vi "5.6.vi"() -> ()   [LabVIEW 2016]
uses:
  <vilib>/sound2/lvsound2.llb/Sound Data Format.ctl
  <vilib>/Analysis/4window.llb/Hamming Window (DBL).vi
  <vilib>/Analysis/2dsp.llb/Real FFT.vi
  <vilib>/Analysis/4window.llb/AllCosWindow (DBL).vi
  <vilib>/sound2/lvsound2.llb/Sound File Info (path).vi
  <vilib>/Analysis/3filter.llb/Butterworth Filter (DBL).vi
  <vilib>/Analysis/NI_AALPro.lvlib
  <vilib>/Analysis/NI_AALBase.lvlib
panel:
  out "count":i32
  out "differentiator output":dbl[](graph)
  out "comparator output":dbl[](graph)
  in  "threshold2":dbl
  out "envelope detector output":dbl[](graph)
  out "All":waveform(dbl)(graph)
  in  "Length":dbl(slide) scale=0.0..1024.0
  out "D":bool
  out "#":bool
  out "0":bool
  out "*":bool
  out "C":bool
  out "9":bool
  out "8":bool
  out "7":bool
  out "B":bool
  out "6":bool
  out "5":bool
  out "4":bool
  out "A":bool
  out "3":bool
  out "2":bool
  out "1":bool
  in  "Threshold":dbl
  out "Sub":waveform(dbl)(graph)
  out "FFT":dbl[](graph)
  out "sampling reate":dbl
  out "sound format":T1={"sample rate (S/s)"=22050.0, "number of channels"=2, "bits per sample"=16}
  in  "Path":path
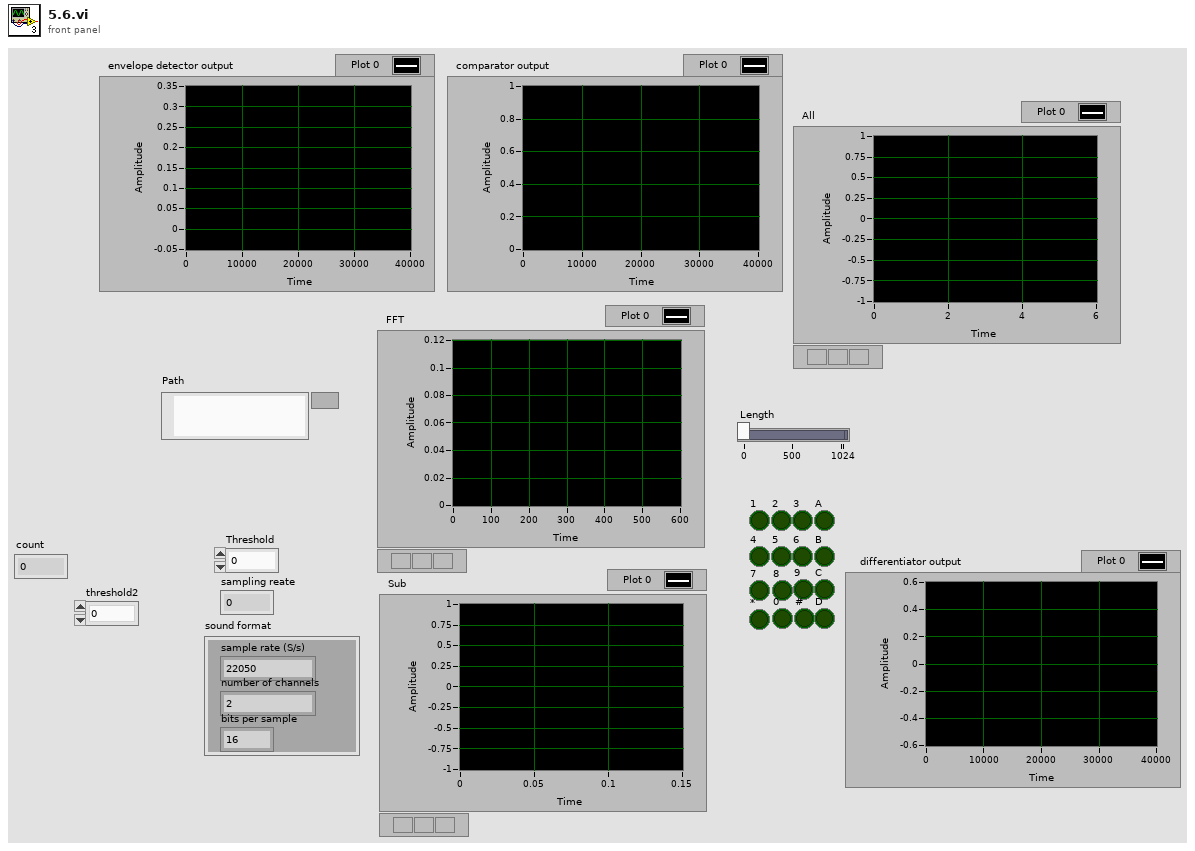
[diagram p1: front panel]
types:
  T1 = typedef "Sound Data Format.ctl" = cluster{"sample rate (S/s)":dbl, "number of channels":i32, "bits per sample":i32}
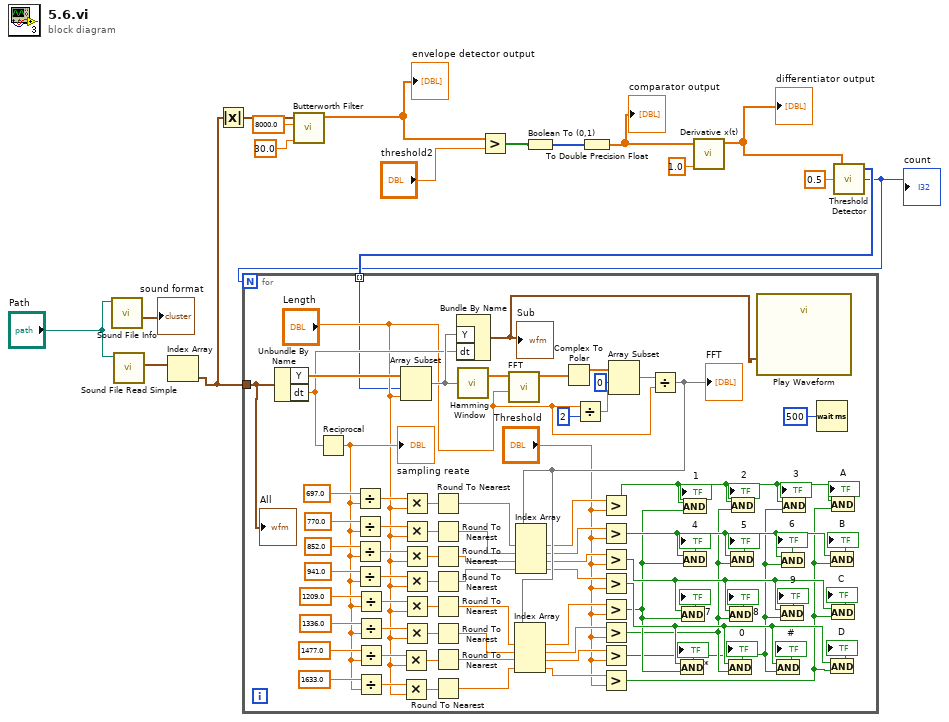
[diagram p0: block diagram]
diagram:
  n1 = call-poly <vilib>:"Sound File Info.vi"("path"="Path") -> ("sound format"=→"sound format":T1)  [unwired: 7 in, 3 out]
  n2 = call <vilib>:"Sound File Read Simple.vi"("path"="Path") -> ("data"=w17:waveform(dbl)[])  [unwired: 7 in, 3 out]
  n3 = Index Array(array=w17) -> (element=w3:waveform(dbl))  [unwired: 1 in]
  n4 = Absolute Value(x=w3) -> (abs(x)=w5:waveform(dbl))
  n5 = call-poly <vilib>:"Butterworth Filter.vi"("low cutoff freq: fl"=30.0, "sampling freq: fs"=8000.0, "X"=w5) -> ("Filtered X"=w13:dbl[])  [unwired: 5 in, 1 out]
  "envelope detector output" <- w13
  n6 = Greater?(x=w13, y="threshold2") -> (0:w11:bool[])
  n7 = Boolean To (0,1)(Boolean=w11) -> (0, 1=w10:i16[])
  n8 = To Double Precision Float(number=w10) -> (double precision float=w9:dbl[])
  "comparator output" <- w9
  n9 = call <vilib>:"Derivative x(t).vi"("dt"=1.0, "X"=w9) -> ("dX/dt"=w7:dbl[])  [unwired: 8 in, 1 out]
  "differentiator output" <- w7
  n10 = call <vilib>:"Threshold Detector.vi"("threshold"=0.5, "X"=w7) -> ("count"=w1:i32, "Indices"=w2:i32[])  [unwired: 1 in, 1 out]
  "count" <- w1
  n11 = for {
    N: w1 -> [_]
    tunnel: w3 -> [w22]
    tunnel: w2 -> [w19] mode=indexing
    n12 = Unbundle By Name(w22) -> ("Y"=w99:dbl[], "dt"=w74:dbl)
    n13 = Reciprocal(x=w74) -> (1/x=w82:dbl)
    "sampling reate" <- w82
    n14 = Divide(x=697.0, y=w82) -> (x/y=w83:dbl)
    n15 = Divide(x=770.0, y=w82) -> (x/y=w84:dbl)
    n16 = Divide(x=852.0, y=w82) -> (x/y=w85:dbl)
    n17 = Divide(x=941.0, y=w82) -> (x/y=w86:dbl)
    n18 = Divide(x=1209.0, y=w82) -> (x/y=w87:dbl)
    n19 = Divide(x=1336.0, y=w82) -> (x/y=w88:dbl)
    n20 = Divide(x=1477.0, y=w82) -> (x/y=w89:dbl)
    n21 = Divide(x=1633.0, y=w82) -> (x/y=w90:dbl)
    n22 = Array Subset(array=w99, index=w19, length="Length") -> (w75:dbl[])
    n23 = Multiply(x=w89, y="Length") -> (x*y=w67:dbl)
    n24 = Multiply(x=w90, y="Length") -> (x*y=w66:dbl)
    n25 = Multiply(x=w83, y="Length") -> (x*y=w73:dbl)
    n26 = Multiply(x=w84, y="Length") -> (x*y=w72:dbl)
    n27 = Multiply(x=w85, y="Length") -> (x*y=w71:dbl)
    n28 = Multiply(x=w86, y="Length") -> (x*y=w70:dbl)
    n29 = Multiply(x=w87, y="Length") -> (x*y=w69:dbl)
    n30 = Multiply(x=w88, y="Length") -> (x*y=w68:dbl)
    n31 = Round To Nearest(number=w73) -> (nearest integer value=w65:dbl)
    n32 = Round To Nearest(number=w72) -> (nearest integer value=w64:dbl)
    n33 = Round To Nearest(number=w71) -> (nearest integer value=w63:dbl)
    n34 = Round To Nearest(number=w70) -> (nearest integer value=w62:dbl)
    n35 = Round To Nearest(number=w69) -> (nearest integer value=w61:dbl)
    n36 = Round To Nearest(number=w68) -> (nearest integer value=w60:dbl)
    n37 = Round To Nearest(number=w67) -> (nearest integer value=w59:dbl)
    n38 = Round To Nearest(number=w66) -> (nearest integer value=w58:dbl)
    n39 = Bundle By Name("Y"=w75, "dt"=w74) -> (w18:waveform(dbl))  [unwired: 1 in]
    "Sub" <- w18
    n40 = call-poly <vilib>:"Hamming Window.vi"("X"=w75) -> ("Windowed X"=w81:dbl[])  [unwired: 1 out]
    n41 = call-poly <vilib>:"FFT.vi"("FFT size"="Length", "X"=w81) -> ("FFT {X}"=w80:cdb[])  [unwired: 8 in, 1 out]
    n42 = Complex To Polar(r * e^(i*theta)=w80) -> (r=w79:dbl[])  [unwired: 1 out]
    n43 = Divide(x="Length", y=2) -> (x/y=w77:dbl)
    n44 = Array Subset(array=w79, index=0, length=w77) -> (w76:dbl[])
    n45 = Divide(x=w76, y="Length") -> (x/y=w57:dbl[])
    "FFT" <- w57
    n46 = Index Array(array=w57, index #1=w61, index #2=w60, index #3=w59, index #4=w58) -> (element #1=w52:dbl, element #2=w51:dbl, element #3=w50:dbl, element #4=w49:dbl)
    n47 = Index Array(array=w57, index #1=w65, index #2=w64, index #3=w63, index #4=w62) -> (element #1=w56:dbl, element #2=w55:dbl, element #3=w54:dbl, element #4=w53:dbl)
    n48 = Greater?(x=w56, y="Threshold") -> (0:w48:bool)
    n49 = Greater?(x=w55, y="Threshold") -> (0:w47:bool)
    n50 = Greater?(x=w54, y="Threshold") -> (0:w46:bool)
    n51 = Greater?(x=w53, y="Threshold") -> (0:w45:bool)
    n52 = Greater?(x=w52, y="Threshold") -> (0:w44:bool)
    n53 = Greater?(x=w51, y="Threshold") -> (0:w43:bool)
    n54 = Greater?(x=w50, y="Threshold") -> (0:w42:bool)
    n55 = Greater?(x=w49, y="Threshold") -> (0:w41:bool)
    n56 = And(x=w45, y=w44) -> (x .and. y?=→"*":bool)
    n57 = And(x=w46, y=w44) -> (x .and. y?=→"7":bool)
    n58 = And(x=w48, y=w44) -> (x .and. y?=→"1":bool)
    n59 = And(x=w47, y=w44) -> (x .and. y?=→"4":bool)
    n60 = And(x=w45, y=w43) -> (x .and. y?=→"0":bool)
    n61 = And(x=w46, y=w43) -> (x .and. y?=→"8":bool)
    n62 = And(x=w47, y=w43) -> (x .and. y?=→"5":bool)
    n63 = And(x=w48, y=w43) -> (x .and. y?=→"2":bool)
    n64 = call "Play Waveform"("Data"=w18) -> ()  [unwired: 18 in, 1 out]
    n65 = And(x=w45, y=w42) -> (x .and. y?=→"#":bool)
    n66 = And(x=w46, y=w42) -> (x .and. y?=→"9":bool)
    n67 = And(x=w47, y=w42) -> (x .and. y?=→"6":bool)
    n68 = And(x=w48, y=w42) -> (x .and. y?=→"3":bool)
    n69 = Wait (ms)(milliseconds to wait=u32 500) -> ()  [unwired: 1 out]
    n70 = And(x=w47, y=w41) -> (x .and. y?=→"B":bool)
    n71 = And(x=w45, y=w41) -> (x .and. y?=→"D":bool)
    n72 = And(x=w48, y=w41) -> (x .and. y?=→"A":bool)
    n73 = And(x=w46, y=w41) -> (x .and. y?=→"C":bool)
    "All" <- w22
  }
